vi "Autonomous.vi"   [LabVIEW 2019]
doc: "This VI starts when autonomous period begins, and will automatically be terminated when it ends. You can carry out timed or sensor driven operations directly to I/O or to subsystems without needing to return to the caller."
uses:
  Framework/Robot Global Data.vi
types:
  T1 = typedef "Single Cmd Info.ctl" = cluster{"Name":string, "CPTM.DataType":variant, "All Control Values Variant":cluster{"Name":string, "Variant Data":variant}[], "icon full":T2, "icon scaled":T2, "Path":path, "Subsystem Color":u32}
  T2 = typedef "imagedata.ctl" = cluster{"image type":i32, "image depth":i32, "image":u8[], "mask":u8[], "colors":u32[], "Rectangle":cluster{"left":i16, "top":i16, "right":i16, "bottom":i16}}
  T3 = cluster{"Robot Backwards":bool, "Path Backwards":bool}
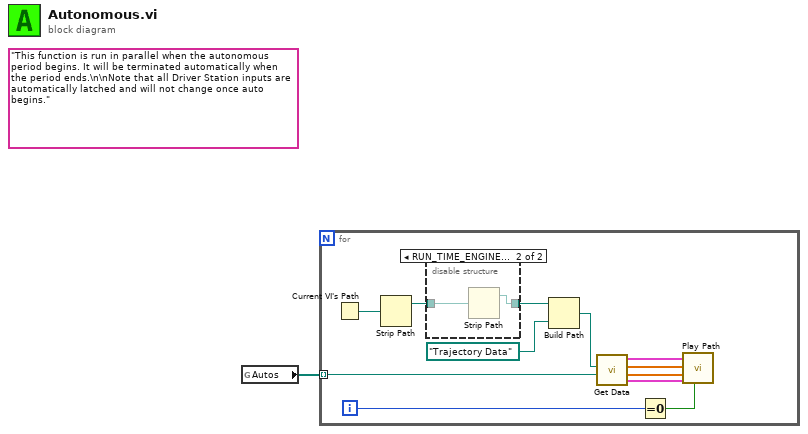
[diagram p0: block diagram]
diagram:
  (unwired) "This function is run in parallel when the autonomous period begins. It will be terminated automatically when the period ends.\n\nNote that all Driver Station inputs are automatically latched and will not change once auto begins."
  n1 = global read "Robot Global Data.vi" "Autos"() -> (w1:path[])
  n2 = for {
    tunnel: w1 -> [w3] mode=indexing
    i -> [w13]
    n3 = Current VI's Path() -> (path=w6:path)
    n4 = Strip Path(path=w6) -> (stripped path=w5:path)  [unwired: 1 out]
    n5 = disable-structure shown="RUN_TIME_ENGINE==True, Default" {
      disable-tunnel: [w14 w15] -> w12
      disable-tunnel: w5 -> [w14 w16]
      frame condition #0 (active) {
      }
      frame condition #1 {
        n6 = Strip Path(path=w16) -> (stripped path=w15:path)  [unwired: 1 out]
      }
    }
    n7 = Build Path(base path=w12, name or relative path=path "Trajectory Data") -> (appended path=w10:path)
    n8 = call "Get Data.vi"("Path Name"=w3, "Path Folder Address"=w10) -> ("Commands"=w2:cluster{"Time (s)":dbl, T1, bool}[], "Angles"=w8:dbl[], "Velocity"=w9:dbl[], "Booleans"=w7:T3)  [unwired: 6 in]
    n9 = Equal To 0?(x=w13) -> (x = 0?=w4:bool)
    n10 = call "Play Path.vi"("Reset Gyro"=w4, "Commands"=w2, "Angles"=w8, "Velocity"=w9, "Booleans"=w7) -> ()  [unwired: 7 in]
  }
